vi "sprawdz_petle_GUI.vi"(7 "Akcja (SET)":T1=enum."SET", 8 "error in (no error)":errorcluster) -> (0 "error out":errorcluster, 2 "Stan":bool)   [LabVIEW 2014]
doc: "Watchdog!\nMonitoruje działanie pętli w której działa jako SET.\nJeżeli zwraca True, znaczy, że pętla działa."
uses:
  Kontrolki/FVGs/FVG akcje podstawowa.ctl
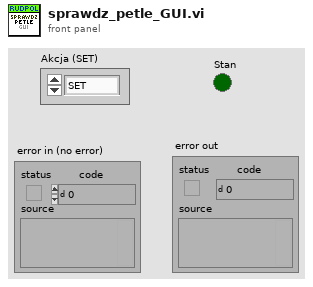
[diagram p1: front panel]
types:
  T1 = typedef "FVG akcje podstawowa.ctl" = enum16{"GET", "SET"}
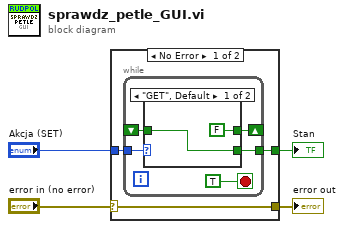
[diagram p0: block diagram]
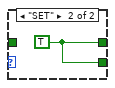
[diagram p2: hidden frame]
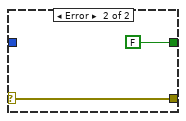
[diagram p3: hidden frame]
diagram:
  n1 = case shown="No Error" "error in (no error)" {
    selector: "error in (no error)" -> [w5 w17]
    tunnel: [w5 w17] -> w3
    tunnel: "Akcja (SET)" -> [w7 _]
    tunnel: [w6 FALSE] -> w1
    frame No Error {
      n2 = while {
        tunnel: w7 -> [w11]
        shift-right: [w10] -> _
        shift-left: _ -> [w9]
        tunnel: [w8] -> w6
        stop <- TRUE stop-if-true
        n3 = case shown="\"GET\", Default" w11 {
          tunnel: [FALSE w15] -> w10
          tunnel: w9 -> [w14 _]
          tunnel: [w14 w15] -> w8
          frame "GET", Default {
          }
          frame "SET" {
            w15 = TRUE
          }
        }
      }
    }
    frame Error {
    }
  }
  "error out" <- w3
  "Stan" <- w1
